vi "Simple Stepper.vi"(1 "Limit":dbl, 2 "Current":dbl, 3 "Target":dbl) -> (0 "coerced(x)":dbl)   [LabVIEW 2013]
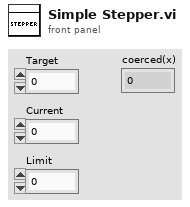
[diagram p1: front panel]
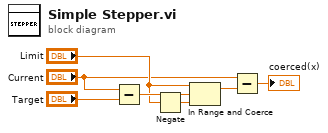
[diagram p0: block diagram]
diagram:
  n1 = Subtract(x="Current", y="Target") -> (x-y=w6:dbl)
  n2 = Negate(x="Limit") -> (-x=w5:dbl)
  n3 = In Range and Coerce(upper limit="Limit", x=w6, lower limit=w5) -> (coerced(x)=w3:dbl)  [unwired: 1 out]
  n4 = Subtract(x="Current", y=w3) -> (x-y=→"coerced(x)":dbl)
